vi "ReadWriteTest (FPGA).vi"() -> ()   [LabVIEW 2009]
panel:
  out "Point Read":cluster{"X":i32, "Y":i32, "Z":i32}
  out "Point Written":cluster{"X":i32, "Y":i32, "Z":i32}
  out "Read Time":u32
  out "Write Time":u32
  out "Numeric":i32
  out "Matched":cluster{"X":bool, "Y":bool, "Z":bool}
  in  "stop":bool
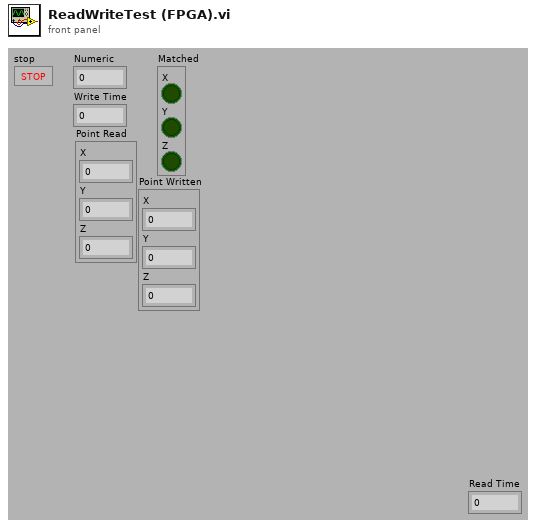
[diagram p1: front panel]
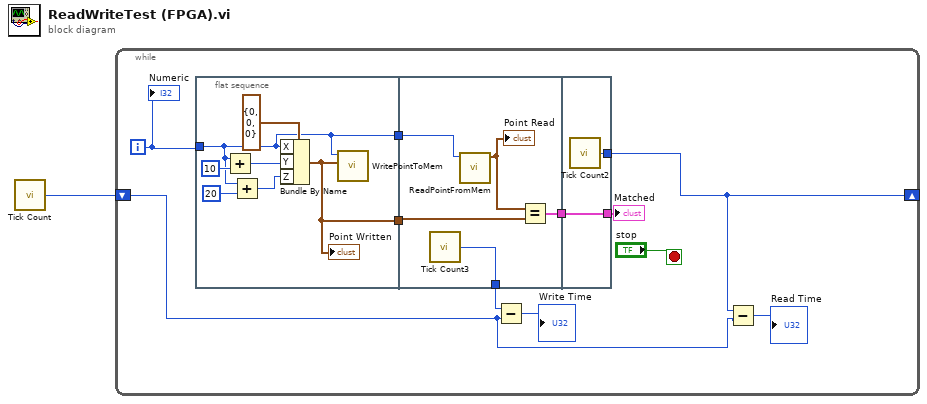
[diagram p0: block diagram]
diagram:
  n1 = call "Tick Count"() -> ("Tick Count(uSec)"=w1:u32)
  n2 = while {
    shift-right: [w3] -> _
    shift-left: w1 -> [w2]
    i -> [w11]
    stop <- "stop" stop-if-true
    n3 = flat-sequence {
      tunnel: w11 -> [w16]
      tunnel: [w16] -> w10
      tunnel: [w18] -> w9
      tunnel: w10 -> [w24]
      tunnel: w9 -> [w22]
      tunnel: [w21] -> w7
      tunnel: [w20] -> w6
      tunnel: [w26] -> w8
      tunnel: w7 -> [w26]
      tunnel: [w25] -> w3
      frame #0 {
        n4 = Add(x=w16, y=10) -> (x+y=w14:i32)
        n5 = Add(x=w16, y=20) -> (x+y=w13:i32)
        n6 = Bundle By Name(cluster=cluster{"X":i32, "Y":i32, "Z":i32} {"X"=0, "Y"=0, "Z"=0} ("Point"), "X"=w16, "Y"=w14, "Z"=w13) -> (w18:cluster{"X":i32, "Y":i32, "Z":i32})
        "Point Written" <- w18
        n7 = call "WritePointToMem.vi"("Point"=w18, "PointNum"=w16) -> ()  [unwired: 10 in]
      }
      frame #1 {
        n8 = call "Tick Count3"() -> ("Tick Count(uSec)"=w20:u32)
        n9 = call "ReadPointFromMem.vi"("PointNum"=w24) -> ("Point"=w23:cluster{"X":i32, "Y":i32, "Z":i32})  [unwired: 10 in]
        "Point Read" <- w23
        n10 = Equal?(x=w23, y=w22) -> (x = y?=w21:cluster{"X":bool, "Y":bool, "Z":bool})
      }
      frame #2 {
        n11 = call "Tick Count2"() -> ("Tick Count(uSec)"=w25:u32)
      }
    }
    n12 = Subtract(x=w6, y=w2) -> (x-y=→"Write Time":u32)
    n13 = Subtract(x=w3, y=w2) -> (x-y=→"Read Time":u32)
    "Matched" <- w8
    "Numeric" <- w11
  }
